vi "DSF.Shared.Configuration.Plugin.Set Custom Parameters.vi"(8 "error in (no error)":errorcluster, 10 "Custom Parameters":variant, 11 "Plugin Configuration in":refnum<class "DSF.Shared.Configuration.Plugin.lvclass">) -> (0 "error out":errorcluster, 3 "Plugin Configuration out":refnum<class "DSF.Shared.Configuration.Plugin.lvclass">)   [LabVIEW 2016, in "DSF.Shared.lvlib" / "DSF.Shared.Configuration.Plugin.lvclass"]
uses:
  DSF.Shared.Configuration.Plugin.lvclass
  DSF.Shared.Configuration.Plugin.lvclass/DSF.Shared.Configuration.Plugin.ctl
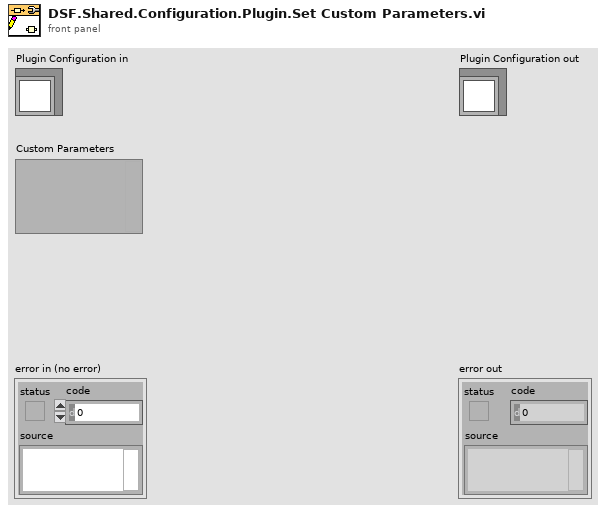
[diagram p1: front panel]
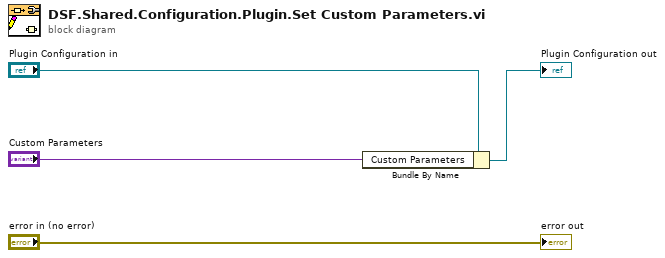
[diagram p0: block diagram]
diagram:
  n1 = Bundle By Name(cluster="Plugin Configuration in", "Custom Parameters"="Custom Parameters") -> (→"Plugin Configuration out":refnum<class "DSF.Shared.Configuration.Plugin.lvclass">)
  "error out" <- "error in (no error)"
